vi "Global - RT Stream Connections.vi"() -> ()   [LabVIEW 2022 SP3]
uses:
  support/Message Queue/Message Cluster.ctl
  support/Message Queue/Message Queue.lvlib
panel:
  in  "RT Writer Stream":refnum<k21>
  in  "UI Writer Stream":refnum<k21>
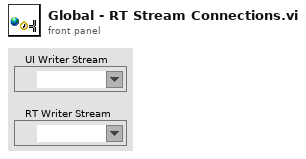
[diagram p1: front panel]
diagram:
